vi "is Pwd Match.vi"(8 "error in (no error)":errorcluster, 9 "password":string, 10 "username":string, 11 "[Data] Userinfo Binary in":refnum<class "[Data] Userinfo Binary.lvclass">) -> (0 "error out":errorcluster, 2 "match?":bool, 3 "[Data] Userinfo Binary out":refnum<class "[Data] Userinfo Binary.lvclass">)   [LabVIEW 2020, in "[Data] Userinfo Binary.lvclass"]
uses:
  [Data] Userinfo Binary.lvclass
  [Data] Userinfo Binary.lvclass/[Data] Userinfo Binary.ctl
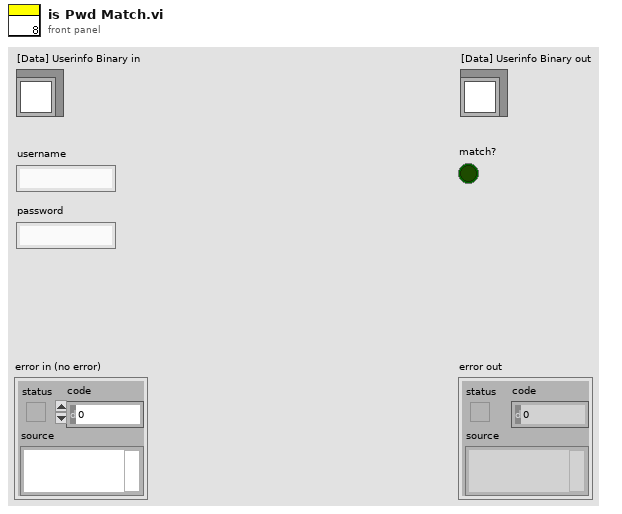
[diagram p1: front panel]
types:
  T1 = typedef "[Data] Userinfo Binary.lvclass/user info.ctl" = cluster{"password":string, "authority":i8, "department":string, "post":string, "remark":string, "create time":timestamp, "last login time":timestamp}
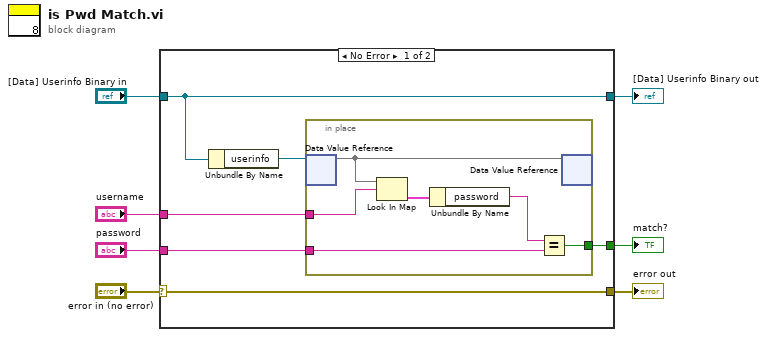
[diagram p0: block diagram]
diagram:
  n1 = case shown="No Error" "error in (no error)" {
    selector: "error in (no error)" -> [w13 w21]
    tunnel: [w13 w21] -> w6
    tunnel: [w12 w20] -> w4
    tunnel: "[Data] Userinfo Binary in" -> [w12 w20]
    tunnel: "username" -> [w11 _]
    tunnel: [w9 _] -> w2
    tunnel: "password" -> [w10 _]
    frame No Error {
      n2 = Unbundle By Name(w12) -> ("userinfo"=w8:refnum<data-value>)
      n3 = in-place {
        in-place-border: w11 -> [w19]
        in-place-border: w10 -> [w17]
        in-place-border: [w15] -> w9
        n4 = in-place-dvr #1(w8) -> (w14:map{string, T1})  [unwired: 1 out]
        n5 = Look In Map(map=w14, key=w19) -> (value=w18:T1)  [unwired: 1 in, 1 out]
        n6 = Unbundle By Name(w18) -> ("password"=w16:string)
        n7 = Equal?(x=w16, y=w17) -> (x = y?=w15:bool)
        n8 = in-place-dvr #1(w14) -> ()  [unwired: 2 out]
      }
    }
    frame Error {
    }
  }
  "error out" <- w6
  "[Data] Userinfo Binary out" <- w4
  "match?" <- w2
